vi "GlobalVariables.vi"() -> ()   [LabVIEW 2009]
panel:
  in  "Sensors to Mask":u32[](array[numeric])=[6, 7, 10, 14, 18, 20, 23] max=23
  in  "DataPath":path=path "C:/OrgCon/ExperimentData"
  in  "Data Collect Stop":bool
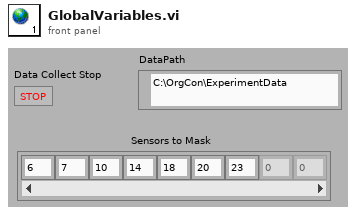
[diagram p1: front panel]
diagram:
